vi "5.vi"() -> ()   [LabVIEW 2018]
panel:
  out "ROJO - EMERGENCIA\nVERDE - ESTABLE":bool
  in  "limite":dbl
  out "sensor de\n temperatura":dbl(slide) scale=0.0..100.0
  in  "millisecond multiple":u32
  in  "stop":bool
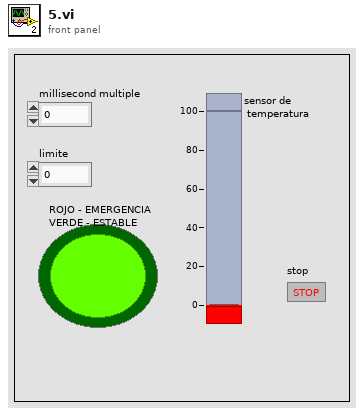
[diagram p1: front panel]
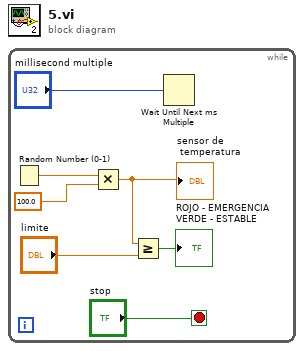
[diagram p0: block diagram]
diagram:
  n1 = while {
    stop <- "stop" stop-if-true
    n2 = Random Number (0-1)() -> (number: 0 to 1=w5:dbl)
    n3 = Multiply(x=w5, y=100.0) -> (x*y=w3:dbl)
    "sensor de\n temperatura" <- w3
    n4 = Greater Or Equal?(x=w3, y="limite") -> (x >= y?=→"ROJO - EMERGENCIA\nVERDE - ESTABLE":bool)
    n5 = Wait Until Next ms Multiple(millisecond multiple="millisecond multiple") -> ()  [unwired: 1 out]
  }
